vi "Condition Finish Create.vi"(4 "Actor Ref":refnum<vi>, 5 "Alias":string, 6 "Creator Attributes":refnum<class "Attributes.lvclass">, 7 "Unified Msg Set":T1, 10 "Queue of Self Attributes":refnum<queue>, 11 "TEMPLATE Actor in":refnum<class "TEMPLATE Actor.lvclass">) -> (0 "Error out":errorcluster, 3 "TEMPLATE Actor out":refnum<class "TEMPLATE Actor.lvclass">)   [LabVIEW 2025, in "TEMPLATE Actor.lvlib" / "TEMPLATE Actor.lvclass"]
uses:
  TEMPLATE Actor.lvclass
  <vilib>/Nathan Davis/jettl/jettl/jettl/Attributes/Attributes/Attributes.lvclass
  <vilib>/Nathan Davis/jettl/jettl/jettl/Actor/Msg Set.ctl
  <vilib>/Nathan Davis/jettl/jettl/jettl/Msg/Msg.lvclass
  TEMPLATE Actor.lvclass/TEMPLATE Actor.ctl
  <vilib>/Nathan Davis/jettl/jettl/jettl/Actor/Actor/Actor.lvclass
  <vilib>/Nathan Davis/jettl/jettl/jettl/Actor/Actor.lvlib
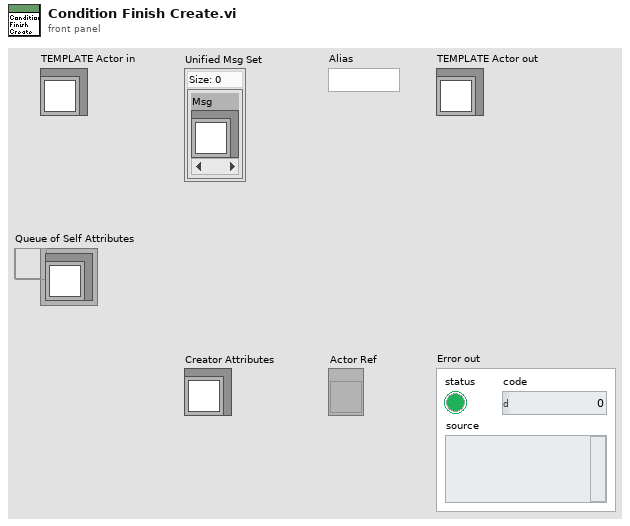
[diagram p1: front panel]
types:
  T1 = typedef "jettl.lvlib/Actor.lvlib/Msg Set.ctl" = set{refnum<class "Msg.lvclass">}
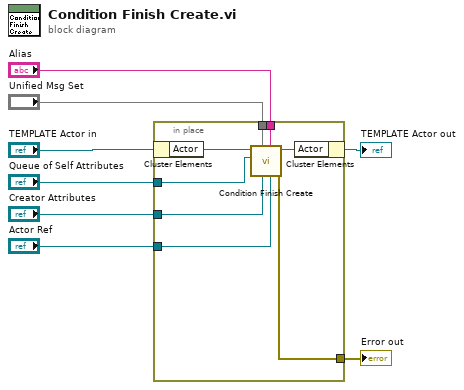
[diagram p0: block diagram]
diagram:
  n1 = in-place {
    in-place-border: "Unified Msg Set" -> [w14]
    in-place-border: "Alias" -> [w13]
    in-place-border: "Creator Attributes" -> [w12]
    in-place-border: "Actor Ref" -> [w11]
    in-place-border: [w10] -> w1
    in-place-border: "Queue of Self Attributes" -> [w9]
    n2 = in-place-cluster #1("TEMPLATE Actor in") -> ("Actor"=w16:refnum<class "Actor.lvclass">)
    n3 = call-dynamic "Condition Finish Create.vi"("Actor Ref"=w11, "Alias"=w13, "Creator Attributes"=w12, "Unified Msg Set"=w14, "Queue of Self Attributes"=w9, "Actor in"=w16) -> ("Error out"=w10:errorcluster, "Actor out"=w15:refnum<class "Actor.lvclass">)  [unwired: 4 in]
    n4 = in-place-cluster #1("Actor"=w15) -> (→"TEMPLATE Actor out":refnum<class "TEMPLATE Actor.lvclass">)
  }
  "Error out" <- w1
